vi "Remove NaN 1D.vi"(10 "Array in":dbl[](array[numeric])) -> (2 "indexes removed":i32[](array[numeric]), 3 "Array out":dbl[](array[numeric]))   [LabVIEW 2009]
panel:
  out "length":i32
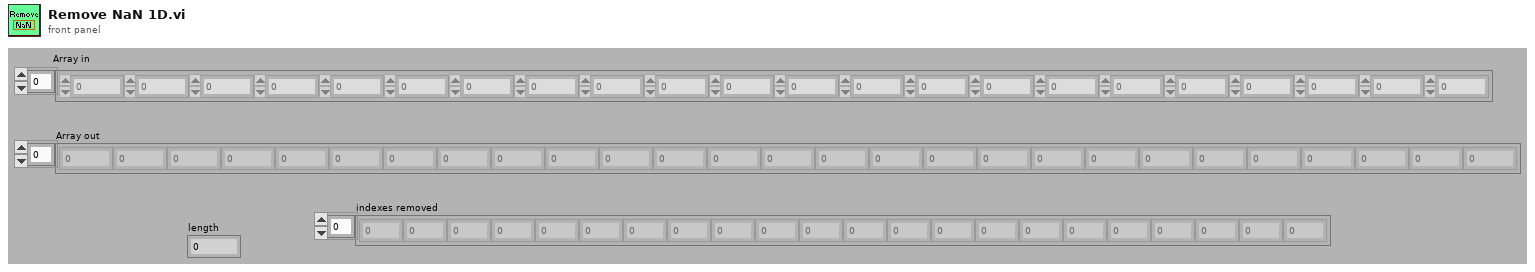
[diagram p1: front panel]
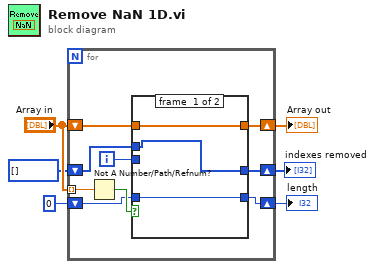
[diagram p0: block diagram]
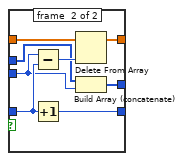
[diagram p2: hidden frame]
diagram:
  n1 = for {
    tunnel: "Array in" -> [w15] mode=indexing
    shift-right: [w12] -> w3
    shift-left: 0 ("length") -> [w13]
    shift-right: [w9] -> w4
    shift-left: "Array in" -> [w10]
    shift-right: [w8] -> w2
    shift-left: i32[] [] -> [w7]
    i -> [w11]
    n2 = Not A Number/Path/Refnum?(number/path/refnum=w15) -> (NaN/Path/Refnum?=w14:bool)
    n3 = case shown="False" w14 {
      tunnel: w10 -> [w17 w26]
      tunnel: w13 -> [w18 w22]
      tunnel: [w18 w24] -> w12
      tunnel: [w17 w25] -> w9
      tunnel: w11 -> [_ w19]
      tunnel: [w16 w21] -> w8
      tunnel: w7 -> [w16 w20]
      frame #0 {
      }
      frame #1 {
        n4 = Subtract(x=w19, y=w22) -> (x-y=w23:i32)
        n5 = Increment(x=w22) -> (x+1=w24:i32)
        n6 = Delete From Array(array=w26, index=w23) -> (array with subset deleted=w25:dbl[])  [unwired: 1 in, 1 out]
        n7 = Build Array (concatenate)(w20, w19) -> (w21:i32[])
      }
    }
  }
  "Array out" <- w4
  "length" <- w3
  "indexes removed" <- w2
